vi "load_waveforms_for_script.vi"(8 "error in (no error)":errorcluster, 10 "Folder containing waveform files":path, 11 "Pulse Generation Script":string="script MyScript\n\t\tRepeat forever \n\t\t\t     Generate mywfm1\n        Generate mywfm2 \n\t\tend repeat \nend script\n") -> (0 "error out":errorcluster, 2 "Array":string[][][](array[string]), 3 "waveform names":string[](array[string]))   [LabVIEW 2011]
uses:
  <vilib>/Utility/file.llb/Read From Spreadsheet File (string).vi
  <vilib>/regexp/Match Regular Expression.xnode
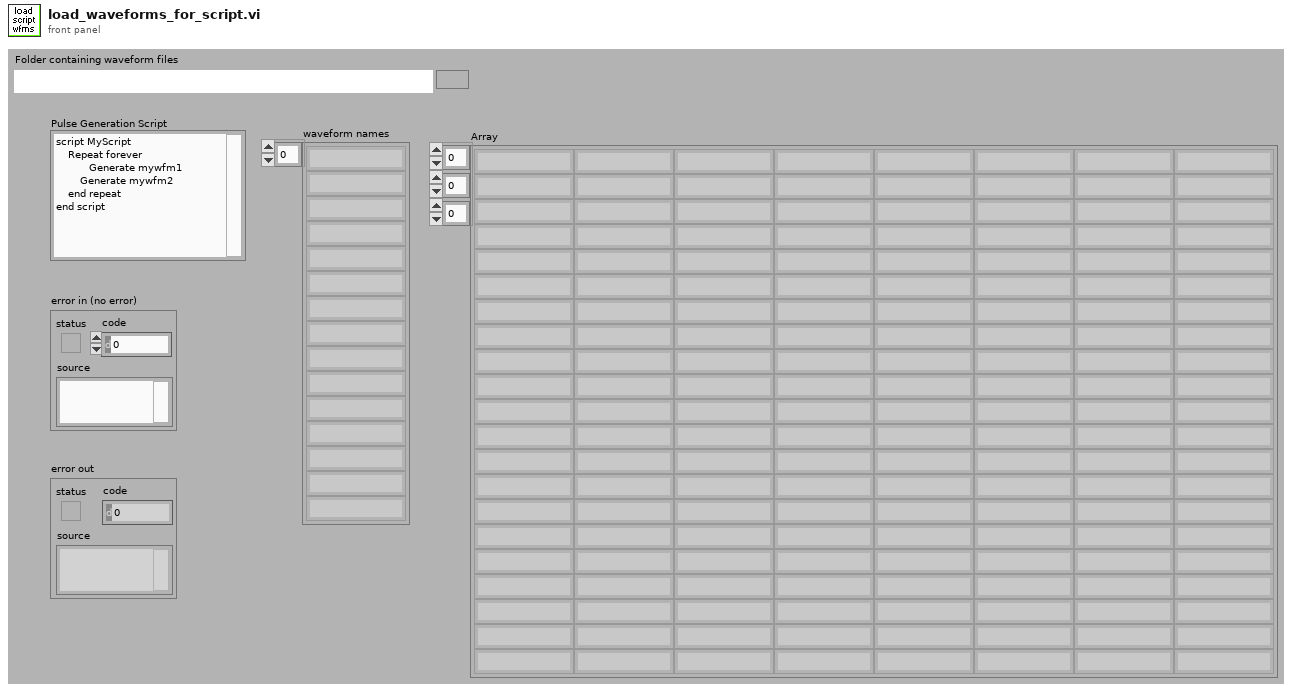
[diagram p1: front panel]
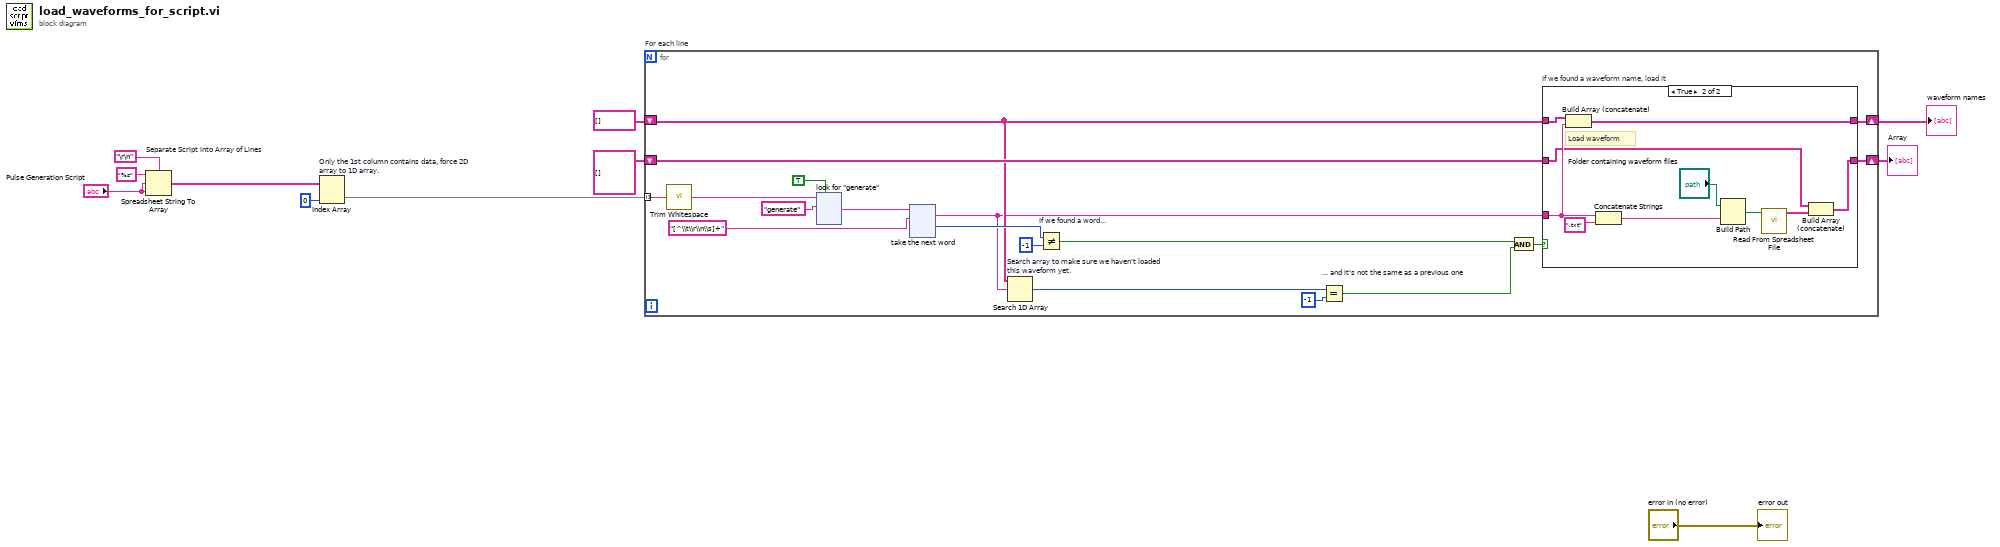
[diagram p0: block diagram]
diagram:
  n1 = Spreadsheet String To Array "Separate Script into Array of Lines"(delimiter (Tab)="\r\n", format string="%s", spreadsheet string="Pulse Generation Script", array type (2D Dbl)="Pulse Generation Script") -> (array=w8:string[][])
  n2 = Index Array "Only the 1st column contains data, force 2D array to 1D array."(array=w8, index (col)=0 ("disabled index (col)")) -> (element=w6:string[])  [unwired: 1 in]
  n3 = for "For each line" {
    tunnel: w6 -> [w29] mode=indexing
    shift-right: [w21] -> w5
    shift-left: string[] [] -> [w18]
    shift-right: [w20] -> w2
    shift-left: string[][][] [] -> [w19]
    n4 = call <vilib>:"Trim Whitespace.vi"("string"=w29) -> ("trimmed string"=w27:string)  [unwired: 1 in]
    n5 = xnode "look for \"generate\""("input string"=w27, "regular expression"="generate", "ignore case? (F)"=TRUE) -> ("after match"=w23:string)  [unwired: 3 in, 4 out]
    n6 = xnode "take the next word"("input string"=w23, "regular expression"="[^\\t\\r\\n\\s]+") -> ("whole match"=w17:string, "offset past match"=w22:i32)  [unwired: 4 in, 3 out]
    n7 = Search 1D Array "Search array to make sure we haven't loaded this waveform yet."(1D array=w18, element=w17) -> (index of element=w12:i32)  [unwired: 1 in]
    n8 = Not Equal? "If we found a word..."(x=w22, y=-1) -> (x != y?=w15:bool)
    n9 = Equal? "... and it's not the same as a previous one"(x=w12, y=-1) -> (x = y?=w14:bool)
    n10 = And(x=w15, y=w14) -> (x .and. y?=w13:bool)
    n11 = case "If we found a waveform name, load it" shown="True" w13 {
      tunnel: w17 -> [_ w35]
      tunnel: [w30 w32] -> w20
      tunnel: [w31 w37] -> w21
      tunnel: w18 -> [w31 w36]
      tunnel: w19 -> [w30 w34]
      frame False {
        # "Don't load anything"
      }
      frame True {
        # "Load waveform"
        n12 = Build Array (concatenate)(w36, w35) -> (w37:string[])
        n13 = Concatenate Strings(w35, ".txt" ("string")) -> (w39:string)
        n14 = Build Path(base path="Folder containing waveform files", name or relative path=w39) -> (appended path=w41:path)
        n15 = call-poly <vilib>:"Read From Spreadsheet File.vi"("file path (dialog if empty)"=w41) -> ("all rows"=w33:string[][])  [unwired: 6 in, 4 out]
        n16 = Build Array (concatenate)(w34, w33) -> (w32:string[][][])
      }
    }
  }
  "waveform names" <- w5
  "Array" <- w2
  "error out" <- "error in (no error)"
